vi "Handle Picture Shortcut Activation.vi"(8 "MenuRef":refnum<k9>, 9 "Container State":T1, 10 "state in":T3={"Draw Options"={"Outer Border Color"=0, "Inner Border Color"=6316128, "Outer Gradient Color"=2565927, "Inner Gradient Color"=16860, "Compass North Pointer Color"=16711680, "Compass Pointer Color 1"=13355429, "Compass Pointer Color 2"=14934973, "Direction Pointer Color"=16765184, "Text Box Outline Color"=13355429, "Text Box Background Color"=14934973, "Scale Color"=16448250, "Text Color"=0, "Draw Gradient"=TRUE, "Draw Rose"=TRUE, "Simple Scale"=TRUE, "Draw Text"=FALSE, "Font Name"="Helvetica", "Angle Units"=enum."Degrees"}} caption="State", 11 "Data":T2 caption="data in") -> ()   [LabVIEW 2017, in "Compass Indicator.xctl"]
uses:
  <vilib>/robotics/Controls/Compass Indicator/Compass Indicator.xctl
  <vilib>/robotics/Controls/Compass Indicator/_Compass Indicator Support Files/Compass State.ctl
  <vilib>/robotics/Controls/Compass Indicator/Compass Picture/Draw Options.ctl
  <vilib>/robotics/Controls/Utilities/Angle Units.ctl
  <vilib>/robotics/Controls/Compass Indicator/_Compass Indicator Support Files/Compass Data.ctl
  <vilib>/_xctls/Container State.ctl
  <vilib>/robotics/Controls/Utilities/NI_Robotics_Control Utilities.lvlib
  <vilib>/robotics/Controls/Compass Indicator/Compass Picture/NI_Robotics_Compass Picture.lvlib
  <vilib>/_xctls/XControlSupport.lvlib
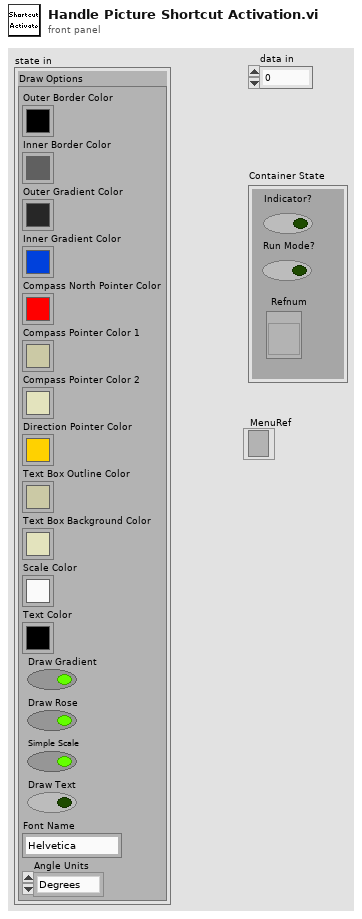
[diagram p1: front panel]
types:
  T1 = typedef "XControlSupport.lvlib/Container State.ctl" = cluster{"Indicator?":bool, "Run Mode?":bool, " Refnum":refnum<vi>}
  T2 = typedef "Compass Indicator.xctl/Compass Data.ctl" = dbl
  T3 = typedef "Compass Indicator.xctl/Compass State.ctl" = cluster{"Draw Options":T4}
  T4 = typedef "NI_Robotics_Compass Picture.lvlib/Draw Options.ctl" = cluster{"Outer Border Color":u32, "Inner Border Color":u32, "Outer Gradient Color":u32, "Inner Gradient Color":u32, "Compass North Pointer Color":u32, "Compass Pointer Color 1":u32, "Compass Pointer Color 2":u32, "Direction Pointer Color":u32, "Text Box Outline Color":u32, "Text Box Background Color":u32, "Scale Color":u32, "Text Color":u32, "Draw Gradient":bool, "Draw Rose":bool, "Simple Scale":bool, "Draw Text":bool, "Font Name":string, "Angle Units":T5}
  T5 = typedef "NI_Robotics_Control Utilities.lvlib/Angle Units.ctl" = enum16{"Radians", "Degrees"}
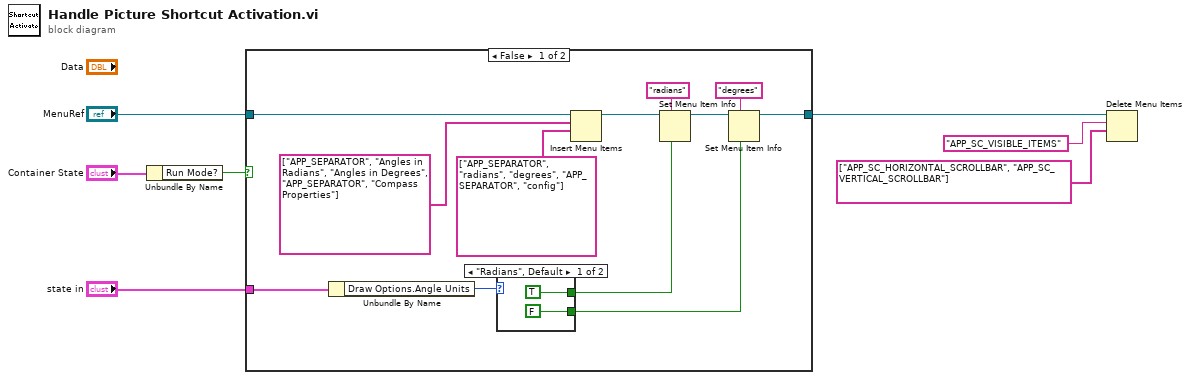
[diagram p0: block diagram]
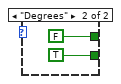
[diagram p2: hidden frame]
diagram:
  n1 = Unbundle By Name("Container State") -> ("Run Mode?"=w4:bool)
  n2 = case shown="False" w4 {
    tunnel: "MenuRef" -> [w10 w24]
    tunnel: "state in" -> [w9 _]
    tunnel: [w8 w24] -> w7
    frame False {
      n3 = Unbundle By Name(w9) -> ("Draw Options.Angle Units"=w17:T5)
      n4 = case shown="\"Radians\", Default" w17 {
        tunnel: [TRUE FALSE] -> w18
        tunnel: [FALSE TRUE] -> w19
        frame "Radians", Default {
        }
        frame "Degrees" {
        }
      }
      n5 = Insert Menu Items(7:string[] ["APP_SEPARATOR", "radians", "degrees", "APP_SEPARATOR", "config"], 8:string[] ["APP_SEPARATOR", "Angles in Radians", "Angles in Degrees", "APP_SEPARATOR", "Compass Properties"], 9:w10) -> (3:w14:refnum<k9>)  [unwired: 3 in, 2 out]
      n6 = Set Menu Item Info(6:w18, 7:"radians" ("item tag"), 11:w14) -> (3:w13:refnum<k9>)  [unwired: 4 in, 1 out]
      n7 = Set Menu Item Info(6:w19, 7:"degrees" ("item tag"), 11:w13) -> (3:w8:refnum<k9>)  [unwired: 4 in, 1 out]
    }
    frame True {
    }
  }
  n8 = Delete Menu Items(7:string[] ["APP_SC_HORIZONTAL_SCROLLBAR", "APP_SC_VERTICAL_SCROLLBAR"], 8:"APP_SC_VISIBLE_ITEMS", 9:w7) -> ()  [unwired: 1 in, 2 out]
